vi "CalculateSynchronous.vi"(6 "calc cache":variant, 7 "Feature":T1, 8 "error in (no error)":errorcluster, 9 "Speed (RPM)":dbl, 11 "Data":waveform(sgl)) -> (0 "error out":errorcluster, 3 "Synchronous [EU RMS]":dbl, 4 "calc cache out":variant)   [LabVIEW 2017, in "AnalysisHelper.lvlib"]
uses:
  <vilib>/addons/InsightCM/Utilities/Analysis/Shared/AnalysisHelper.lvlib
  <vilib>/addons/InsightCM/Utilities/Analysis/Shared/controls/Feature.ctl
  <vilib>/addons/InsightCM/Utilities/Analysis/Shared/controls/AmplitudeScale.ctl
  <vilib>/addons/InsightCM/Utilities/Analysis/Vibration/VibrationAnalysisFunctions.lvlib
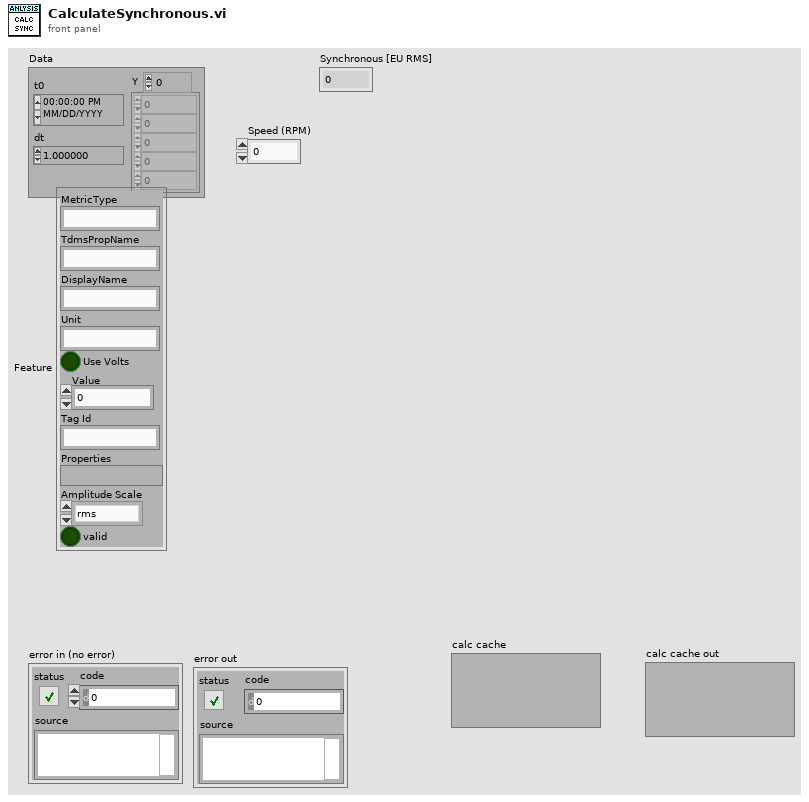
[diagram p1: front panel]
types:
  T1 = typedef "AnalysisHelper.lvlib/Feature.ctl" = cluster{"MetricType":string, "TdmsPropName":string, "DisplayName":string, "Unit":string, "Use Volts":bool, "Value":dbl, "Tag Id":string, "Properties":variant, "Amplitude Scale":T2, "valid":bool}
  T2 = typedef "AnalysisHelper.lvlib/AmplitudeScale.ctl" = enum16{"rms", "peak", "pk-pk"}
  T3 = typedef "svc_Spectrum Info.ctl" = cluster{"channel name":string, "description":string, "x-axis units":T4, "spectral info":cluster{"spectrum type":T5, "linear/dB":enum16{"linear", "dB"}, "window":u16, "window size":i32, "FFT size":i32}, "engineering units":T6, "custom label":string, "dB reference [EU]":dbl, "peak units":enum16{"rms", "peak", "peak-peak"}, "weighting filter":T7, "spectral density?":bool, "unit label":string, "spectrum skewed?":bool, "complimentary spectrum units":T8}
  T4 = typedef "svc_X-Axis Units.ctl" = u16
  T5 = typedef "svc_Spectrum Type.ctl" = enum16{"FFT Spectrum [complex]", "Amplitude [Magnitude]", "Power [Magnitude^2]", "Cross Spectrum [complex]", "Frequency Response [Complex]"}
  T6 = typedef "svc_Engineering Units Text Ring.ctl" = u16
  T7 = typedef "svc_Weighting Filter Text Ring.ctl" = u16
  T8 = typedef "svc_Complimentary Spectrum Units.ctl" = enum16{"none", "radians", "degrees", "cycles", "imaginary"}
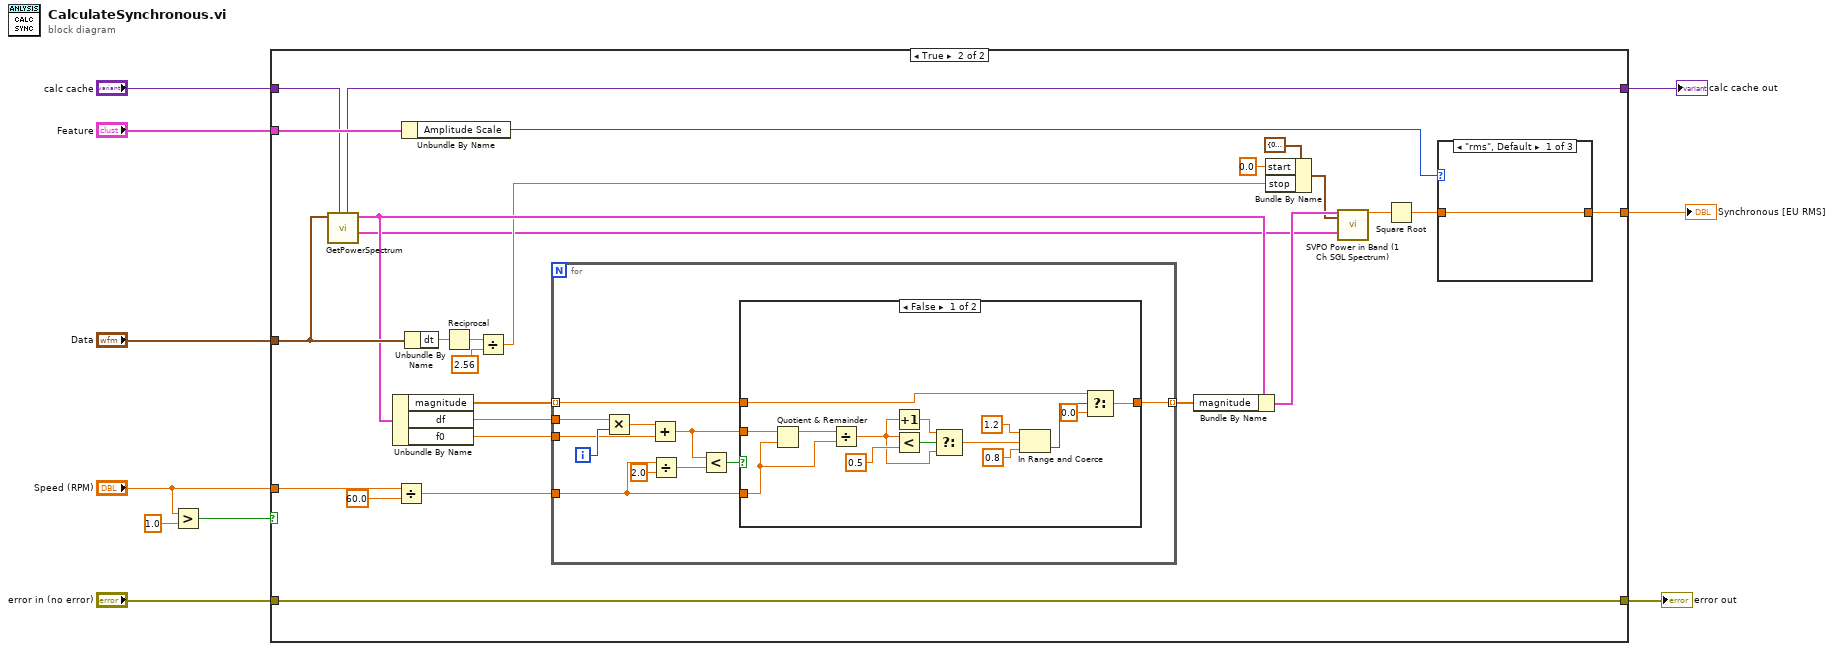
[diagram p0: block diagram]
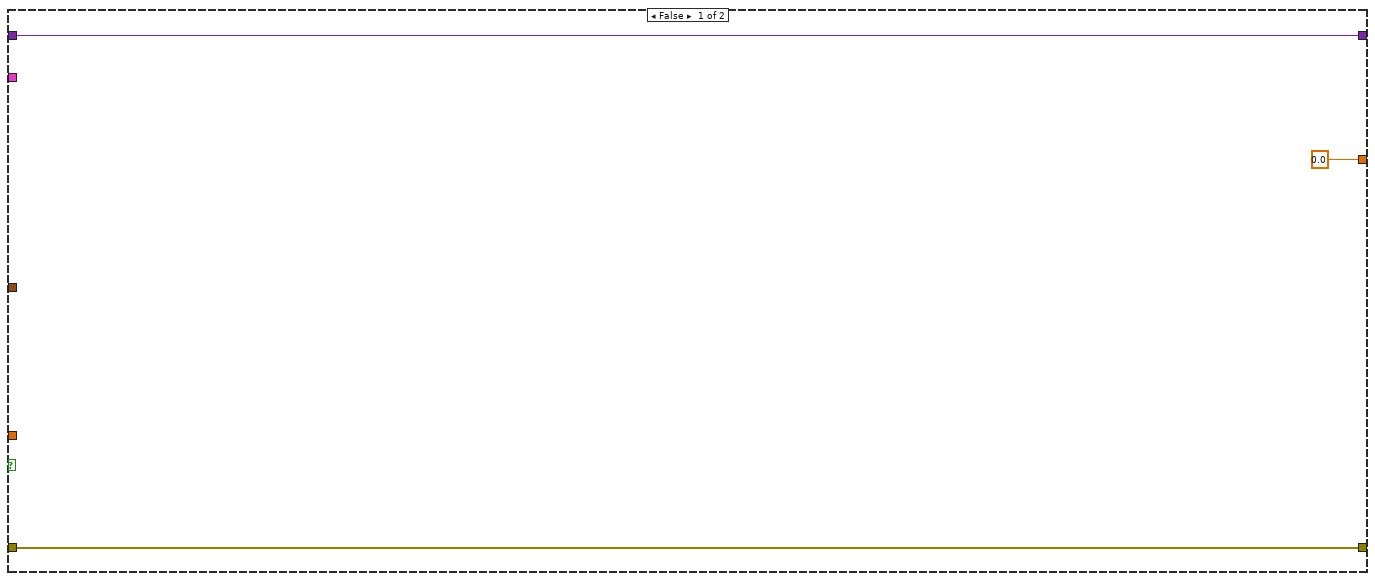
[diagram p2: hidden frame]
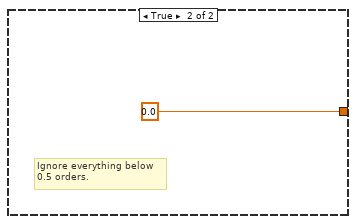
[diagram p3: hidden frame]
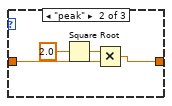
[diagram p4: hidden frame]
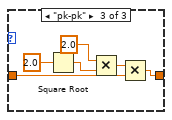
[diagram p5: hidden frame]
diagram:
  n1 = Greater?(x="Speed (RPM)", y=1.0) -> (0:w3:bool)
  n2 = case shown="True" w3 {
    tunnel: "Speed (RPM)" -> [_ w16]
    tunnel: "Data" -> [_ w38]
    tunnel: "error in (no error)" -> [w12 w28]
    tunnel: "Feature" -> [_ w27]
    tunnel: [0.0 w26] -> w7
    tunnel: "calc cache" -> [w11 w20]
    tunnel: [w12 w28] -> w5
    tunnel: [w11 w18] -> w1
    frame False {
    }
    frame True {
      n3 = call <vilib>:"GetPowerSpectrum.vi"("calc cache"=w20, "Waveform"=w38) -> ("spectrum info"=w22:T3, "power spectrum [EU^2 rms]"=w34:cluster{"f0":dbl, "df":dbl, "magnitude":sgl[]}, "calc cache out"=w18:variant)  [unwired: 7 in]
      n4 = Unbundle By Name(w34) -> ("magnitude"=w32:sgl[], "df"=w39:dbl, "f0"=w17:dbl)
      n5 = Divide(x=w16, y=60.0) -> (x/y=w14:dbl)
      n6 = Unbundle By Name(w27) -> ("Amplitude Scale"=w25:T2)
      n7 = Unbundle By Name(w38) -> ("dt"=w37:dbl)
      n8 = Reciprocal(x=w37) -> (1/x=w36:dbl)
      n9 = Divide(x=w36, y=2.56) -> (x/y=w29:dbl)
      n10 = for {
        tunnel: w32 -> [w41] mode=indexing
        tunnel: w39 -> [w50]
        tunnel: w17 -> [w48]
        tunnel: w14 -> [w40]
        tunnel: [w43] -> w33 mode=indexing
        i -> [w49]
        n11 = Multiply(x=w50, y=w49) -> (x*y=w47:dbl)
        n12 = Add(x=w47, y=w48) -> (x+y=w42:dbl)
        n13 = Divide(x=w40, y=2.0) -> (x/y=w44:dbl)
        n14 = Less?(x=w42, y=w44) -> (x < y?=w46:bool)
        n15 = case shown="False" w46 {
          tunnel: [w52 0.0 ("y")] -> w43
          tunnel: w42 -> [w64 _]
          tunnel: w41 -> [w53 _]
          tunnel: w40 -> [w62 _]
          frame False {
            n16 = Quotient & Remainder(x=w64, y=w62) -> (x-y*floor(x/y)=w63:dbl)  [unwired: 1 out]
            n17 = Divide(x=w63, y=w62) -> (x/y=w58:dbl)
            n18 = Increment(x=w58) -> (x+1=w59:dbl)
            n19 = Less?(x=w58, y=0.5) -> (x < y?=w60:bool)
            n20 = Select(t=w59, s=w60, f=w58) -> (s? t:f=w55:dbl)
            n21 = In Range and Coerce(upper limit=1.2, x=w55, lower limit=0.8) -> (In Range?=w54:bool)  [unwired: 1 out]
            n22 = Select(t=w53, s=w54, f=0.0) -> (s? t:f=w52:dbl)
          }
          frame True {
            # "Ignore everything below\n0.5 orders."
          }
        }
      }
      n23 = Bundle By Name(cluster=w34, "magnitude"=w33) -> (w24:cluster{"f0":dbl, "df":dbl, "magnitude":sgl[]})
      n24 = Bundle By Name(cluster=cluster{"start":dbl, "stop":dbl} {"start"=0.0, "stop"=1000.0} ("range"), "start"=0.0, "stop"=w29) -> (w23:cluster{"start":dbl, "stop":dbl})
      n25 = call <vilib>:"SVPO Power in Band (1 Ch SGL Spectrum).vi"("spectrum [EU^2 rms]"=w24, "range"=w23, "spectrum info"=w22) -> ("power in band [EU^2 rms]"=w21:dbl)  [unwired: 16 in]
      n26 = Square Root(x=w21) -> (sqrt(x)=w19:dbl)
      n27 = case shown="\"rms\", Default" w25 {
        tunnel: w19 -> [w66 w70 w76]
        tunnel: [w66 w69 w75] -> w26
        frame "rms", Default {
        }
        frame "peak" {
          n28 = Square Root(x=sgl 2.0) -> (sqrt(x)=w68:sgl)
          n29 = Multiply(x=w68, y=w70) -> (x*y=w69:dbl)
        }
        frame "pk-pk" {
          n30 = Square Root(x=sgl 2.0) -> (sqrt(x)=w72:sgl)
          n31 = Multiply(x=sgl 2.0, y=w72) -> (x*y=w73:sgl)
          n32 = Multiply(x=w73, y=w76) -> (x*y=w75:dbl)
        }
      }
    }
  }
  "Synchronous [EU RMS]" <- w7
  "error out" <- w5
  "calc cache out" <- w1
